vi "Unflatten Pixmap 32-bit pixmap.vi"(10 "image data":T1) -> (0 "1-bit pixmap":bool[][](array[boolean]), 1 "4-bit pixmap":u8[][](array[numeric]), 2 "8-bit pixmap":u8[][](array[numeric]), 3 "24-bit pixmap":u32[][](array[numeric]) format="%x", 4 "colors":u32[](array[numeric]), 5 "32-bit pixmap":u32[][](array[numeric]) format="%x", 6 "mask":u8[](array[numeric]), 7 "top left":cluster{"x":i16, "y":i16})   [LabVIEW 2021, in "Picture2D.lvlib"]
doc: "Converts a cluster of image data into a 2D array."
uses:
  Picture2D/Picture2D.lvlib
  <vilib>/picture/picture.llb/imagedata.ctl
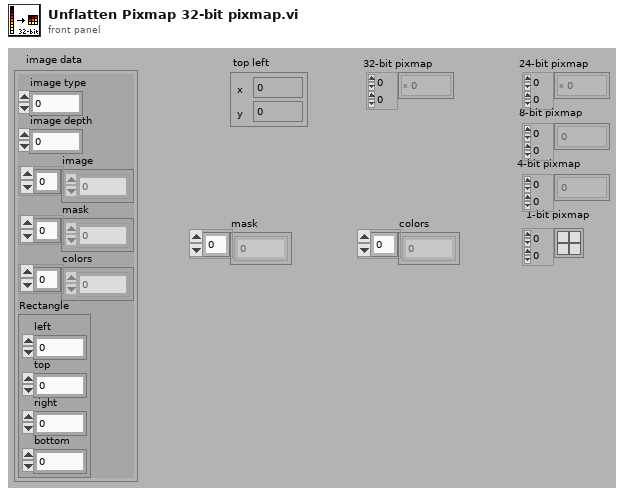
[diagram p1: front panel]
types:
  T1 = typedef "imagedata.ctl" = cluster{"image type":i32, "image depth":i32, "image":u8[], "mask":u8[], "colors":u32[], "Rectangle":cluster{"left":i16, "top":i16, "right":i16, "bottom":i16}}
  T2 = cluster{"left":i16, "top":i16, "right":i16, "bottom":i16}
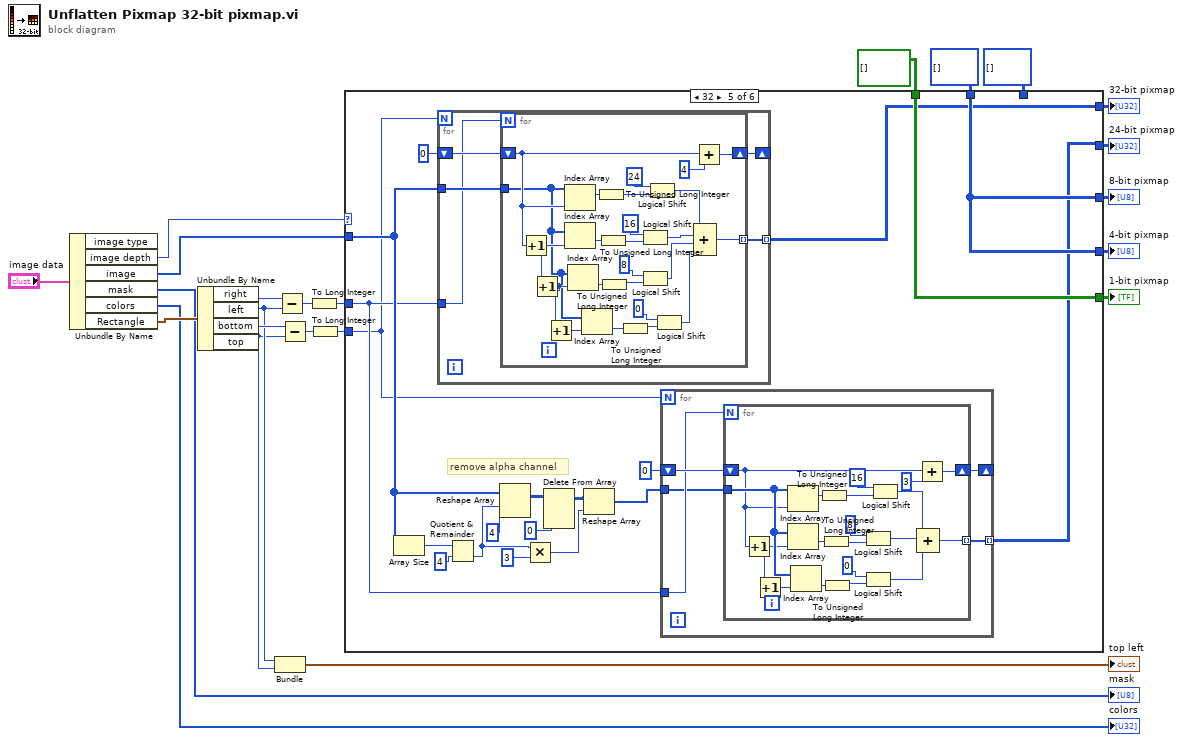
[diagram p0: block diagram]
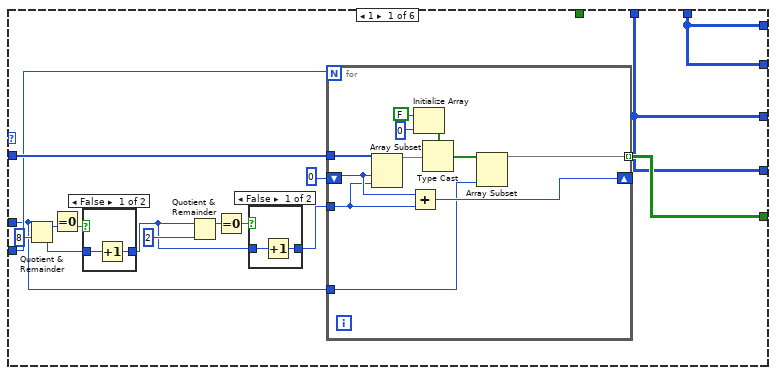
[diagram p2: hidden frame]
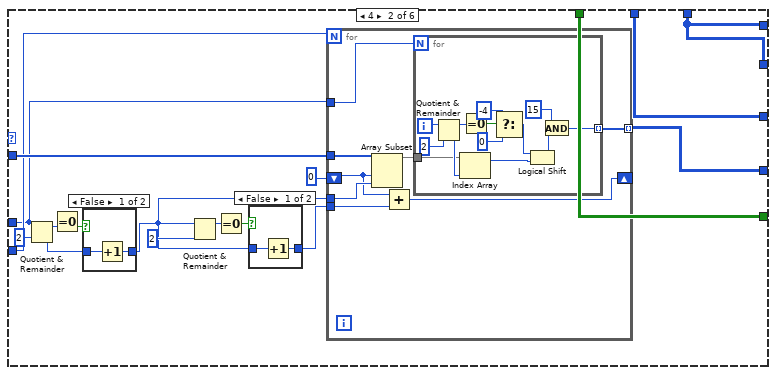
[diagram p5: hidden frame]
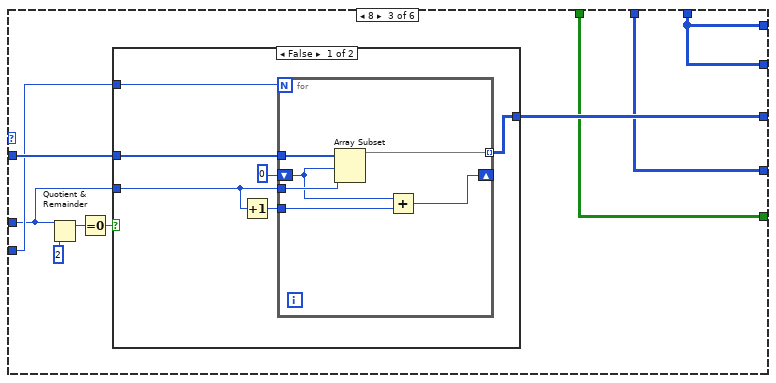
[diagram p8: hidden frame]
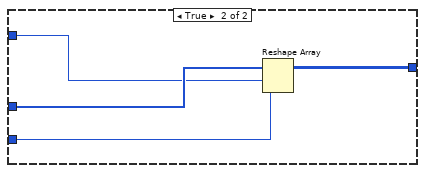
[diagram p9: hidden frame]
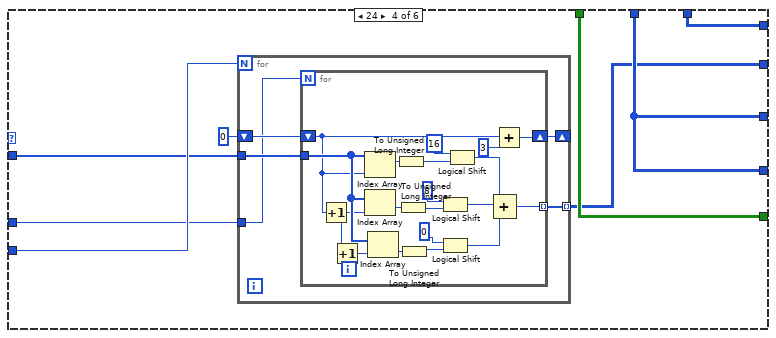
[diagram p10: hidden frame]
diagram:
  n1 = Unbundle By Name("image data") -> ("image depth"=w4:i32, "image"=w5:u8[], "mask"=→"mask":u8[], "colors"=→"colors":u32[], "Rectangle"=w8:T2)  [unwired: 1 out]
  n2 = Unbundle By Name(w8) -> ("right"=w23:i16, "left"=w11:i16, "bottom"=w22:i16, "top"=w10:i16)
  n3 = Bundle("left"=w11, "top"=w10) -> (→"top left":cluster{"left":i16, "top":i16})  [unwired: 1 in]
  n4 = Subtract(x=w23, y=w11) -> (x-y=w21:i16)
  n5 = Subtract(x=w22, y=w10) -> (x-y=w20:i16)
  n6 = To Long Integer(number=w21) -> (32bit integer=w2:i32)
  n7 = To Long Integer(number=w20) -> (32bit integer=w1:i32)
  n8 = case shown="32" w4 {
    tunnel: w5 -> [w39 w73 w108 w130 w163 _]
    tunnel: w2 -> [w27 w60 w105 w131 w161 _]
    tunnel: w1 -> [w32 w66 w106 w132 w160 _]
    tunnel: [w34 w59 w102 w134 w177 w233] -> w19
    tunnel: u8[][] [] ("4-bit pixmap") -> [w33 w67 w103 w133 w176 w232]
    tunnel: [w33 w58 w103 w133 w176 w232] -> w17
    tunnel: bool[][] [] ("1-bit pixmap") -> [_ w59 w102 w134 w177 w233]
    tunnel: [w33 w67 w107 w133 w176 w232] -> w15
    tunnel: [w24 w57 w101 w129 w173 w231] -> w14
    tunnel: u32[][] [] ("24-bit pixmap") -> [w24 w57 w101 w127 _ w231]
    tunnel: [w24 w57 w101 w127 w174 w231] -> w3
    frame 1 {
      n9 = Quotient & Remainder(x=w27, y=8) -> (x-y*floor(x/y)=w30:i32, floor(x/y)=w28:i32)
      n10 = Equal To 0?(x=w30) -> (x = 0?=w29:bool)
      n11 = case shown="False" w29 {
        tunnel: w28 -> [w41 w42]
        tunnel: [w40 w42] -> w26
        frame False {
          n12 = Increment(x=w41) -> (x+1=w40:i32)
        }
        frame True {
        }
      }
      n13 = Quotient & Remainder(x=w26, y=2) -> (x-y*floor(x/y)=w37:i32)  [unwired: 1 out]
      n14 = Equal To 0?(x=w37) -> (x = 0?=w36:bool)
      n15 = case shown="False" w36 {
        tunnel: w26 -> [w44 w45]
        tunnel: [w43 w45] -> w25
        frame False {
          n16 = Increment(x=w44) -> (x+1=w43:i32)
        }
        frame True {
        }
      }
      n17 = for {
        N: w32 -> [_]
        tunnel: w39 -> [w56]
        shift-right: [w51] -> _
        shift-left: 0 -> [w55]
        tunnel: w25 -> [w46]
        tunnel: [w48] -> w34 mode=indexing
        tunnel: w27 -> [w49]
        n18 = Array Subset(array=w56, index=w55, length=w46) -> (w47:u8[])
        n19 = Add(x=w55, y=w46) -> (x+y=w51:i32)
        n20 = Initialize Array(FALSE, 0) -> (w54:bool[])
        n21 = Type Cast(type=w54, x=w47) -> (*(type *) &x=w50:bool[])
        n22 = Array Subset(array=w50, length=w49) -> (w48:bool[])  [unwired: 1 in]
      }
    }
    frame 4 {
      n23 = Quotient & Remainder(x=w60, y=2) -> (x-y*floor(x/y)=w64:i32, floor(x/y)=w62:i32)
      n24 = Equal To 0?(x=w64) -> (x = 0?=w63:bool)
      n25 = case shown="False" w63 {
        tunnel: w62 -> [w75 w76]
        tunnel: [w74 w76] -> w61
        frame False {
          n26 = Increment(x=w75) -> (x+1=w74:i32)
        }
        frame True {
        }
      }
      n27 = Quotient & Remainder(x=w61, y=2) -> (x-y*floor(x/y)=w71:i32)  [unwired: 1 out]
      n28 = Equal To 0?(x=w71) -> (x = 0?=w70:bool)
      n29 = case shown="False" w70 {
        tunnel: w61 -> [w78 w79]
        tunnel: [w77 w79] -> w68
        frame False {
          n30 = Increment(x=w78) -> (x+1=w77:i32)
        }
        frame True {
        }
      }
      n31 = for {
        N: w66 -> [_]
        tunnel: w73 -> [w87]
        shift-right: [w83] -> _
        shift-left: 0 -> [w85]
        tunnel: w61 -> [w86]
        tunnel: w68 -> [w84]
        tunnel: w60 -> [w80]
        tunnel: [w81] -> w58 mode=indexing
        n32 = Array Subset(array=w87, index=w85, length=w86) -> (w82:u8[])
        n33 = Add(x=w85, y=w84) -> (x+y=w83:i32)
        n34 = for {
          N: w80 -> [_]
          tunnel: w82 -> [w94]
          tunnel: [w95] -> w81 mode=indexing
          i -> [w99]
          n35 = Quotient & Remainder(x=w99, y=2) -> (x-y*floor(x/y)=w92:i32, floor(x/y)=w98:i32)
          n36 = Index Array(array=w94, index=w98) -> (element=w93:u8)
          n37 = Equal To 0?(x=w92) -> (x = 0?=w91:bool)
          n38 = Select(t=i8 -4, s=w91, f=i8 0) -> (s? t:f=w88:i8)
          n39 = Logical Shift(y=w88, x=w93) -> (x << y=w96:u8)
          n40 = And(x=u8 15, y=w96) -> (x .and. y?=w95:u8)
        }
      }
    }
    frame 8 {
      n41 = Quotient & Remainder(x=w105, y=2) -> (x-y*floor(x/y)=w109:i32)  [unwired: 1 out]
      n42 = Equal To 0?(x=w109) -> (x = 0?=w104:bool)
      n43 = case shown="False" w104 {
        tunnel: w108 -> [w116 w125]
        tunnel: [w113 w126] -> w107
        tunnel: w106 -> [w115 w124]
        tunnel: w105 -> [w112 w123]
        frame False {
          n44 = Increment(x=w112) -> (x+1=w111:i32)
          n45 = for {
            N: w115 -> [_]
            tunnel: w116 -> [w122]
            shift-right: [w119] -> _
            shift-left: 0 -> [w120]
            tunnel: w112 -> [w121]
            tunnel: [w118] -> w113 mode=indexing
            tunnel: w111 -> [w117]
            n46 = Array Subset(array=w122, index=w120, length=w121) -> (w118:u8[])
            n47 = Add(x=w120, y=w117) -> (x+y=w119:i32)
          }
        }
        frame True {
          n48 = Reshape Array(w125, w124, w123) -> (w126:u8[][])
        }
      }
    }
    frame 24 {
      n49 = for {
        N: w132 -> [_]
        tunnel: w131 -> [w135]
        tunnel: w130 -> [w139]
        tunnel: [w138] -> w129 mode=indexing
        shift-right: [w136] -> _
        shift-left: 0 -> [w137]
        n50 = for {
          N: w135 -> [_]
          tunnel: w139 -> [w158]
          tunnel: [w148] -> w138 mode=indexing
          shift-right: [w146] -> w136
          shift-left: w137 -> [w145]
          n51 = Increment(x=w145) -> (x+1=w144:i32)
          n52 = Increment(x=w144) -> (x+1=w157:i32)
          n53 = Index Array(array=w158, index=w145) -> (element=w151:u8)
          n54 = Index Array(array=w158, index=w144) -> (element=w143:u8)
          n55 = Index Array(array=w158, index=w157) -> (element=w152:u8)
          n56 = To Unsigned Long Integer(number=w151) -> (unsigned 32bit integer=w141:u32)
          n57 = To Unsigned Long Integer(number=w143) -> (unsigned 32bit integer=w154:u32)
          n58 = To Unsigned Long Integer(number=w152) -> (unsigned 32bit integer=w153:u32)
          n59 = Logical Shift(y=i8 8, x=w154) -> (x << y=w150:u32)
          n60 = Logical Shift(y=i8 0, x=w153) -> (x << y=w149:u32)
          n61 = Logical Shift(y=i8 16, x=w141) -> (x << y=w140:u32)
          n62 = Add(x=w145, y=3) -> (x+y=w146:i32)
          n63 = Compound Arithmetic op=ADD(w140, w150, w149) -> (w148:u32)
        }
      }
    }
    frame 32 {
      # "remove alpha channel"
      n64 = Array Size(array=w163) -> (size(s)=w172:i32)
      n65 = for {
        N: w160 -> [_]
        tunnel: w161 -> [w202]
        tunnel: w163 -> [w206]
        tunnel: [w205] -> w174 mode=indexing
        shift-right: [w203] -> _
        shift-left: 0 -> [w204]
        n66 = for {
          N: w202 -> [_]
          tunnel: w206 -> [w207]
          tunnel: [w222] -> w205 mode=indexing
          shift-right: [w220] -> w203
          shift-left: w204 -> [w219]
          n67 = Increment(x=w219) -> (x+1=w218:i32)
          n68 = Increment(x=w218) -> (x+1=w209:i32)
          n69 = Increment(x=w209) -> (x+1=w210:i32)
          n70 = Index Array(array=w207, index=w219) -> (element=w225:u8)
          n71 = Index Array(array=w207, index=w218) -> (element=w217:u8)
          n72 = Index Array(array=w207, index=w209) -> (element=w226:u8)
          n73 = Index Array(array=w207, index=w210) -> (element=w213:u8)
          n74 = To Unsigned Long Integer(number=w225) -> (unsigned 32bit integer=w215:u32)
          n75 = To Unsigned Long Integer(number=w217) -> (unsigned 32bit integer=w228:u32)
          n76 = To Unsigned Long Integer(number=w226) -> (unsigned 32bit integer=w227:u32)
          n77 = To Unsigned Long Integer(number=w213) -> (unsigned 32bit integer=w212:u32)
          n78 = Logical Shift(y=i8 16, x=w228) -> (x << y=w224:u32)
          n79 = Logical Shift(y=i8 8, x=w227) -> (x << y=w223:u32)
          n80 = Logical Shift(y=i8 24, x=w215) -> (x << y=w214:u32)
          n81 = Logical Shift(y=i8 0, x=w212) -> (x << y=w208:u32)
          n82 = Add(x=w219, y=4) -> (x+y=w220:i32)
          n83 = Compound Arithmetic op=ADD(w214, w224, w223, w208) -> (w222:u32)
        }
      }
      n84 = Quotient & Remainder(x=w172, y=4) -> (floor(x/y)=w168:i32)  [unwired: 1 out]
      n85 = Reshape Array(w163, w168, 4 ("dimension size")) -> (w170:u8[][])
      n86 = Multiply(x=w168, y=3) -> (x*y=w166:i32)
      n87 = Delete From Array(array=w170, index (col)=0 ("dimension size")) -> (array with subset deleted=w165:u8[][])  [unwired: 2 in, 1 out]
      n88 = Reshape Array(w165, w166) -> (w162:u8[])
      n89 = for {
        N: w160 -> [_]
        tunnel: w161 -> [w179]
        tunnel: w162 -> [w178]
        tunnel: [w182] -> w173 mode=indexing
        shift-right: [w180] -> _
        shift-left: 0 -> [w181]
        n90 = for {
          N: w179 -> [_]
          tunnel: w178 -> [w201]
          tunnel: [w191] -> w182 mode=indexing
          shift-right: [w189] -> w180
          shift-left: w181 -> [w188]
          n91 = Increment(x=w188) -> (x+1=w187:i32)
          n92 = Increment(x=w187) -> (x+1=w200:i32)
          n93 = Index Array(array=w201, index=w188) -> (element=w194:u8)
          n94 = Index Array(array=w201, index=w187) -> (element=w186:u8)
          n95 = Index Array(array=w201, index=w200) -> (element=w195:u8)
          n96 = To Unsigned Long Integer(number=w194) -> (unsigned 32bit integer=w184:u32)
          n97 = To Unsigned Long Integer(number=w186) -> (unsigned 32bit integer=w197:u32)
          n98 = To Unsigned Long Integer(number=w195) -> (unsigned 32bit integer=w196:u32)
          n99 = Logical Shift(y=i8 8, x=w197) -> (x << y=w193:u32)
          n100 = Logical Shift(y=i8 0, x=w196) -> (x << y=w192:u32)
          n101 = Logical Shift(y=i8 16, x=w184) -> (x << y=w183:u32)
          n102 = Add(x=w188, y=3) -> (x+y=w189:i32)
          n103 = Compound Arithmetic op=ADD(w183, w193, w192) -> (w191:u32)
        }
      }
    }
    frame Default {
    }
  }
  "1-bit pixmap" <- w19
  "4-bit pixmap" <- w17
  "8-bit pixmap" <- w15
  "24-bit pixmap" <- w14
  "32-bit pixmap" <- w3
